vi "ParsePN_SN.vi"(8 "error in (no error)":errorcluster, 9 "SerialNumber":string, 10 "Revision":string, 11 "PartNumber":string) -> (0 "error out":errorcluster, 3 "description":string)   [LabVIEW 2021]
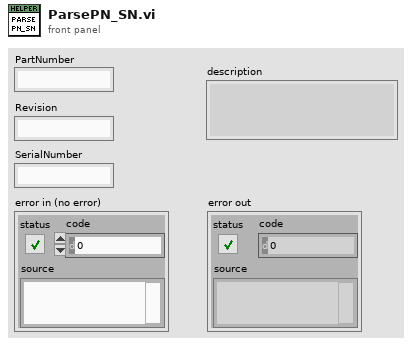
[diagram p1: front panel]
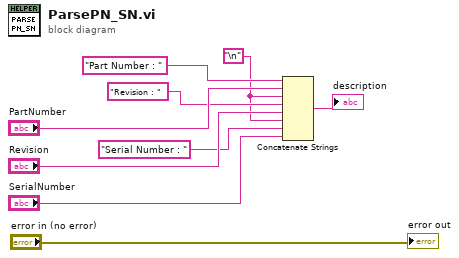
[diagram p0: block diagram]
diagram:
  w1 = "\n"
  n1 = Concatenate Strings("Part Number : " ("string"), "PartNumber", w1, "Revision : " ("string"), "Revision", w1, "Serial Number : " ("string"), "SerialNumber") -> (→"description":string)
  "error out" <- "error in (no error)"
